vi "BRig_dataMTrig_Solenoid_s_L.vi"() -> (2 "output_Solenoid_s_L":i32)   [LabVIEW 2014]
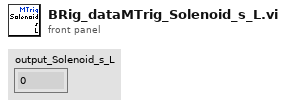
[diagram p1: front panel]
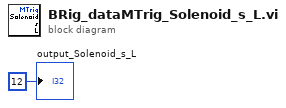
[diagram p0: block diagram]
diagram:
  "output_Solenoid_s_L" <- 12 ("output_iBlock")
